vi "lab session 1.1.vi"() -> ()   [LabVIEW 2020]
panel:
  out "Product":dbl
  out "Sum":dbl
  in  "y":dbl
  in  "x":dbl
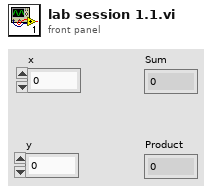
[diagram p1: front panel]
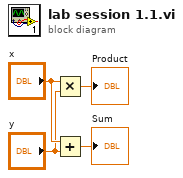
[diagram p0: block diagram]
diagram:
  n1 = Multiply(x="x", y="y") -> (x*y=→"Product":dbl)
  n2 = Add(x="x", y="y") -> (x+y=→"Sum":dbl)
